vi "Logfile_Data_Line.vi"(2 "System Monitor Cluster":T1={"Time"=[], "LI1CH1"=[], "LI1CH2"=[], "LI2CH1"=[], "LI2CH2"=[], "LI3CH1"=[], "LI3CH2"=[], "Field"=[], "N_Level"=[], "H_Level"=[], "Heat_370"=[], "Sorb_Heat"=[], "Still_Heat"=[], "Capacity"=[], "Loss"=[], "Magnet_Temperature"=[], "Lam_Pressure"=[], "Lam_NValve"=[], "370-T1"=[], "370-T2"=[], "370-T3"=[], "370-T4"=[], "370-T5"=[], "370-R1"=[], "370-R2"=[], "370-R3"=[], "370-R4"=[], "370-R5"=[], "372-T1"=[], "372-T2"=[], "372-T3"=[], "372-T4"=[], "372-T5"=[], "372-T6"=[], "372-R1"=[], "372-R2"=[], "372-R3"=[], "372-R4"=[], "372-R5"=[], "372-R6"=[], "Nada"=[nan], "K2440_Res"=[], "K2440_Current"=[], "VTI_Heater"=[], "VTI_NValve"=[], "LS340_Heater"=[], "K6221_Amplitude"=[], "K6221_Frequency"=[], "Cond_Pressure"=[], "Still_Pressure"=[], "FP_Out_Pressure"=[], "Dump_Pressure"=[], "V1"=[], "V2"=[], "V4"=[], "V5"=[], "V9"=[], "Forepump"=[], "Compressor"=[], "K6221_Offset"=[], "BoxTemp"=[], "By"=[], "Bz"=[], "Phi"=[], "heater-recond (%)"=[], "Dewar Pressure "=[], "JT-SP-Control"=[], "350 T1"=[], "350 T2"=[], "350 T3"=[], "350 T4"=[], "350 R1"=[], "350 R2"=[], "350 R3"=[], "350 R4"=[], "Angle"=[], "VTI CH1"=[], "VTI CH2"=[], "VTI CH3"=[]}) -> (0 "Data Line":string)   [LabVIEW 2018]
uses:
  Global/Global Variables/System Monitor Cluster.ctl
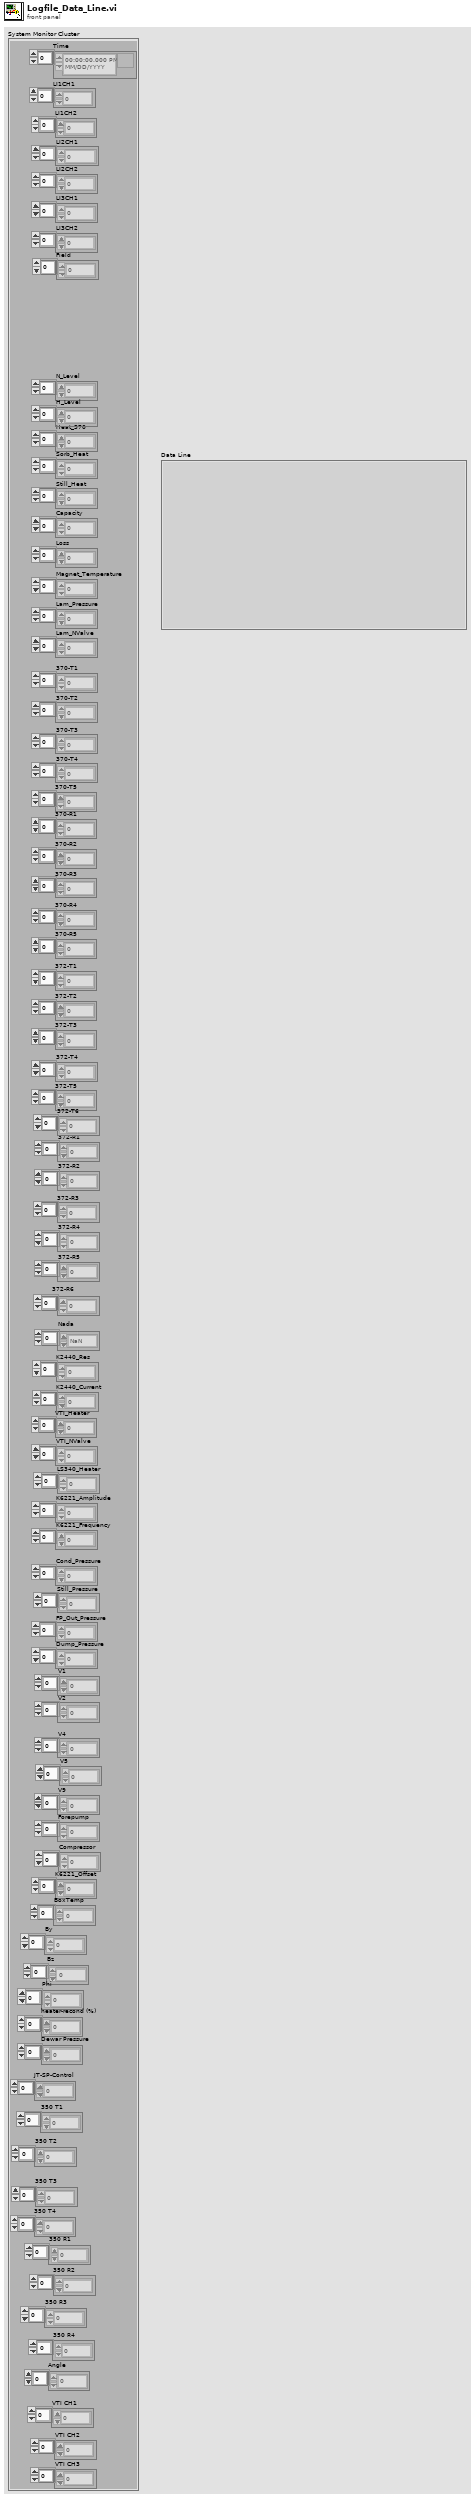
[diagram p1: front panel]
types:
  T1 = typedef "System Monitor Cluster.ctl" = cluster{"Time":timestamp[], "LI1CH1":dbl[], "LI1CH2":dbl[], "LI2CH1":dbl[], "LI2CH2":dbl[], "LI3CH1":dbl[], "LI3CH2":dbl[], "Field":dbl[], "N_Level":dbl[], "H_Level":dbl[], "Heat_370":dbl[], "Sorb_Heat":dbl[], "Still_Heat":dbl[], "Capacity":dbl[], "Loss":dbl[], "Magnet_Temperature":dbl[], "Lam_Pressure":dbl[], "Lam_NValve":dbl[], "370-T1":dbl[], "370-T2":dbl[], "370-T3":dbl[], "370-T4":dbl[], "370-T5":dbl[], "370-R1":dbl[], "370-R2":dbl[], "370-R3":dbl[], "370-R4":dbl[], "370-R5":dbl[], "372-T1":dbl[], "372-T2":dbl[], "372-T3":dbl[], "372-T4":dbl[], "372-T5":dbl[], "372-T6":dbl[], "372-R1":dbl[], "372-R2":dbl[], "372-R3":dbl[], "372-R4":dbl[], "372-R5":dbl[], "372-R6":dbl[], "Nada":dbl[], "K2440_Res":dbl[], "K2440_Current":dbl[], "VTI_Heater":dbl[], "VTI_NValve":dbl[], "LS340_Heater":dbl[], "K6221_Amplitude":dbl[], "K6221_Frequency":dbl[], "Cond_Pressure":dbl[], "Still_Pressure":dbl[], "FP_Out_Pressure":dbl[], "Dump_Pressure":dbl[], "V1":dbl[], "V2":dbl[], "V4":dbl[], "V5":dbl[], "V9":dbl[], "Forepump":dbl[], "Compressor":dbl[], "K6221_Offset":dbl[], "BoxTemp":dbl[], "By":dbl[], "Bz":dbl[], "Phi":dbl[], "heater-recond (%)":dbl[], "Dewar Pressure ":dbl[], "JT-SP-Control":dbl[], "350 T1":dbl[], "350 T2":dbl[], "350 T3":dbl[], "350 T4":dbl[], "350 R1":dbl[], "350 R2":dbl[], "350 R3":dbl[], "350 R4":dbl[], "Angle":dbl[], "VTI CH1":dbl[], "VTI CH2":dbl[], "VTI CH3":dbl[]}
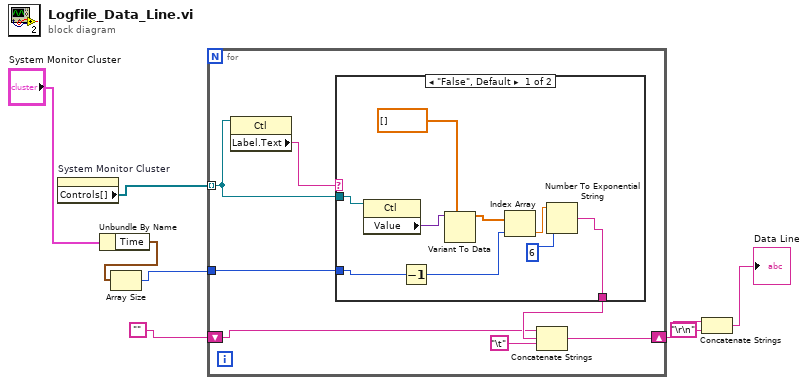
[diagram p0: block diagram]
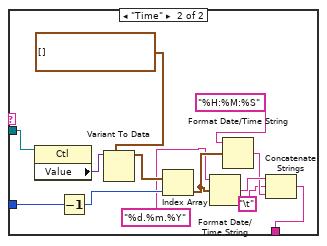
[diagram p2: hidden frame]
diagram:
  n1 = property on="System Monitor Cluster" class="Clust (strict)"() -> ("Controls[]"=w8:refnum<vi>[])  [unwired: 2 in, 2 out]
  n2 = Unbundle By Name("System Monitor Cluster") -> ("Time"=w2:timestamp[])
  n3 = Array Size(array=w2) -> (size(s)=w1:i32)
  n4 = for {
    tunnel: w8 -> [w15] mode=indexing
    shift-right: [w10] -> w6
    shift-left: "" -> [w11]
    tunnel: w1 -> [w9]
    n5 = property class="Ctl"(reference=w15) -> ("Label.Text"=w14:string)  [unwired: 1 in, 2 out]
    n6 = case shown="\"False\", Default" w14 {
      tunnel: w15 -> [w24 w37]
      tunnel: [w16 w31] -> w13
      tunnel: w9 -> [w20 w30]
      frame "False", Default {
        n7 = property class="Ctl"(reference=w24) -> ("Value"=w22:variant)  [unwired: 1 in, 2 out]
        n8 = Decrement(x=w20) -> (x-1=w19:i32)
        n9 = Variant To Data(type=dbl[] [], Variant=w22) -> (data=w21:dbl[])  [unwired: 1 in, 1 out]
        n10 = Index Array(array=w21, index=w19) -> (element=w18:dbl)
        n11 = Number To Exponential String(number=w18, 3:6) -> (E-format string=w16:string)  [unwired: 2 in]
      }
      frame "Time" {
        n12 = property class="Ctl"(reference=w37) -> ("Value"=w35:variant)  [unwired: 1 in, 2 out]
        n13 = Decrement(x=w30) -> (x-1=w29:i32)
        n14 = Variant To Data(type=timestamp[] [], Variant=w35) -> (data=w34:timestamp[])  [unwired: 1 in, 1 out]
        n15 = Index Array(array=w34, index=w29) -> (element=w32:timestamp)
        n16 = Format Date/Time String(time format string (%c)="%d.%m.%Y", seconds (now)=w32) -> (date/time string=w27:string)  [unwired: 1 in]
        n17 = Format Date/Time String(time format string (%c)="%H:%M:%S", seconds (now)=w32) -> (date/time string=w26:string)  [unwired: 1 in]
        n18 = Concatenate Strings(w27, "\t", w26) -> (w31:string)
      }
    }
    n19 = Concatenate Strings(w11, w13, "\t") -> (w10:string)
  }
  n20 = Concatenate Strings(w6, "\r\n") -> (→"Data Line":string)
